vi "Initialize Front Panel.vi"(8 "error in (no error)":errorcluster, 11 "View Manager in":refnum<class "View Manager.lvclass">=refnum) -> (0 "error out":errorcluster, 3 "View Manager out":refnum<class "View Manager.lvclass">)   [LabVIEW 2017, in "View Manager.lvlib" / "View Manager.lvclass"]
doc: "<License>\nCopyright © 2017 Composed Systems, LLC | All rights reserved\nwww.composed.io\n\nAuthor: Ethan Stern <ethan.stern@composed.io>\n\nThis software is provided \"AS IS\" WITHOUT WARRANTIES, either express or implied, AND IS FOR EDUCATIONAL PURPOSES ONLY.\n</License>"
uses:
  View Manager.lvclass
  <vilib>/gpm_packages/@cs/mva-viewable/Source/IViewManager/IViewManager/IViewManager.lvclass
  <vilib>/gpm_packages/@cs/mva-viewable/Source/IViewable/IViewable Messages/Insert Front Panel Msg/Insert Front Panel Msg.lvclass
  C:/Program Files/National Instruments/LabVIEW 2017/vi.lib/gpm_packages/@cs/mva-viewable/Source/IViewable/IViewable/IViewable.lvclass
  C:/Program Files/National Instruments/LabVIEW 2017/vi.lib/gpm_packages/@cs/mva-viewable/Source/ActorEvents/IEventAggregator/IEventAggregator.lvclass
  C:/Program Files/National Instruments/LabVIEW 2017/vi.lib/gpm_packages/@cs/mva-core/Source/IObserver/IObserver/IObserver.lvclass
  C:/Program Files/National Instruments/LabVIEW 2017/vi.lib/ActorFramework/Actor/Actor.lvclass
  <vilib>/gpm_packages/@cs/mva-viewable/Source/IViewable/ProtectedSubpanel/ProtectedSubpanel.lvclass
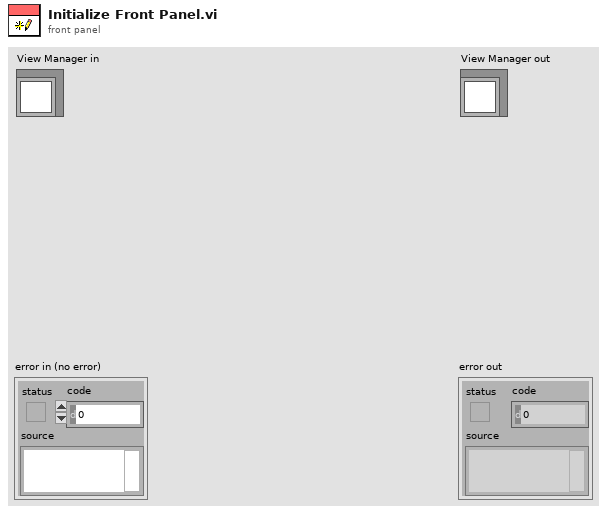
[diagram p1: front panel]
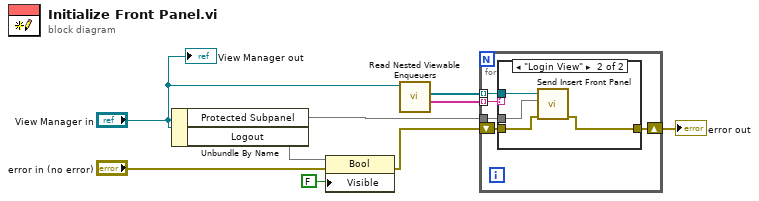
[diagram p0: block diagram]
diagram:
  n1 = Unbundle By Name("View Manager in") -> ("Protected Subpanel"=w4, "Logout"=w1)
  n2 = property on="Property Node" class="Bool"(reference=w1, error in="error in (no error)", "Visible"=FALSE) -> (error out=w3:errorcluster)  [unwired: 1 out]
  n3 = call <vilib>:"Read Nested Viewable Enqueuers.vi"("IViewManager in"="View Manager in") -> ("Viewable Names"=w5:string[], "Nested Viewable Enqueuers"=w6:refnum<class "Message Enqueuer.lvclass">[])  [unwired: 9 in]
  n4 = for {
    tunnel: w6 -> [w14] mode=indexing
    tunnel: w5 -> [w13] mode=indexing
    tunnel: w4 -> [w12]
    shift-right: [w10] -> w2
    shift-left: w3 -> [w11]
    n5 = case shown="\"Login View\"" w13 {
      tunnel: w14 -> [_ w19]
      tunnel: w12 -> [_ w18]
      tunnel: w11 -> [w15 w17]
      tunnel: [w15 w16] -> w10
      frame "False", Default {
      }
      frame "Login View" {
        n6 = call <vilib>:"Send Insert Front Panel.vi"("error in (no error)"=w17, "Protected Subpanel"=w18, "Message Enqueuer"=w19) -> ("error out"=w16:errorcluster)  [unwired: 7 in, 1 out]
      }
    }
  }
  "error out" <- w2
  "View Manager out" <- "View Manager in"
